vi "Create (Config).vi"(8 "error in (no error)":errorcluster, 10 "Scaling Config":refnum<class "Scaling.lvclass">) -> (0 "error out":errorcluster, 3 "VolatusScaling out":refnum<class "Scaling.lvclass">)   [LabVIEW 2020, in "VolatusData.lvlib" / "Scaling.lvclass"]
uses:
  Scaling.lvclass
  Scaling.lvclass/Scaling.ctl
  VolatusConfig/Scaling/Scaling.lvclass
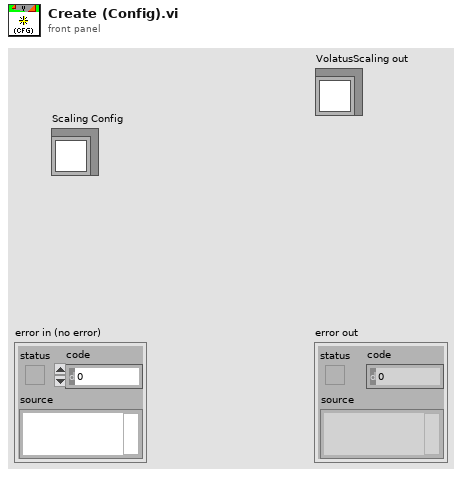
[diagram p1: front panel]
types:
  T1 = typedef "VolatusConfig.lvlib/Scale Type.ctl" = enum16{"None", "Sensor", "Polynomial", "Threshold", "Invert Bool"}
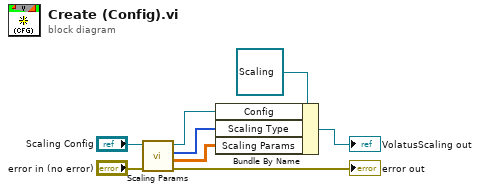
[diagram p0: block diagram]
diagram:
  n1 = call "Scaling Params.vi"("error in (no error)"="error in (no error)", "Scaling in"="Scaling Config") -> ("error out"=→"error out":errorcluster, "Scale Params"=w5:dbl[][], "Scale Types"=w4:T1[], "Scaling out"=w3:refnum<class "Scaling.lvclass">)  [unwired: 6 in]
  n2 = Bundle By Name(cluster=refnum<class "Scaling.lvclass"> refnum ("VolatusScaling in"), "Config"=w3, "Scaling Type"=w4, "Scaling Params"=w5) -> (→"VolatusScaling out":refnum<class "Scaling.lvclass">)
